vi "RSZVB Get Converter Port Assignment.vi"(8 "error in (no error)":errorcluster {"code" format="%.0x"}, 10 "Port (1)":i32=1, 11 "VISA resource name":refnum<visa-resource-name>) -> (0 "error out":errorcluster {"code" format="%.0x"}, 2 "Serial Number":string, 3 "VISA resource name out":refnum<visa-resource-name>)   [LabVIEW 2011]
doc: "This VI returns the assigned R&S ZCxxx converter to port no. <Port>\n\nRemote-control command(s):\n[SENSe<Ch>:]CONVerter:ASSign<Port>?"
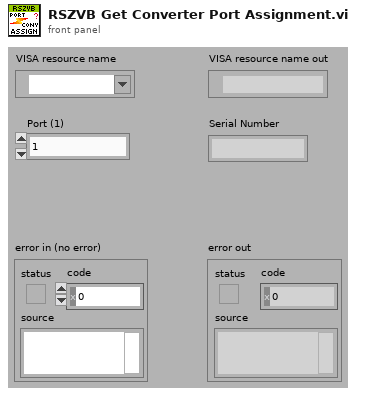
[diagram p1: front panel]
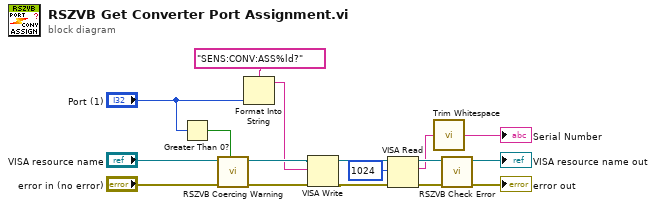
[diagram p0: block diagram]
diagram:
  n1 = Greater Than 0?(x="Port (1)") -> (x > 0?=w11:bool)
  n2 = call "RSZVB Coercing Warning.vi"("In Range?"=w11, "error in (no error)"="error in (no error)", "VISA session"="VISA resource name") -> ("error out"=w9:errorcluster, "dup VISA session"=w10:refnum<visa-resource-name>)  [unwired: 7 in]
  n3 = Format Into String(format string="SENS:CONV:ASS%ld?", "Port (1)") -> (resulting string=w8:string)  [unwired: 2 in, 1 out]
  n4 = VISA Write(VISA resource name=w10, write buffer=w8, error in (no error)=w9) -> (VISA resource name out=w14:refnum<visa-resource-name>, error out=w13:errorcluster)  [unwired: 1 out]
  n5 = VISA Read(VISA resource name=w14, byte count=u32 1024 ("byte count (0)"), error in (no error)=w13) -> (VISA resource name out=w17:refnum<visa-resource-name>, read buffer=w2:string, error out=w16:errorcluster)  [unwired: 1 out]
  n6 = call <vilib>:"Trim Whitespace.vi"("string"=w2) -> ("trimmed string"=→"Serial Number":string)  [unwired: 1 in]
  n7 = call "RSZVB Check Error.vi"("error in (no error)"=w16, "VISA session"=w17) -> ("error out"=→"error out":errorcluster, "dup VISA session"=→"VISA resource name out":refnum<visa-resource-name>)  [unwired: 8 in]
